vi "Sequence.AddVariables.vi"(8 "error in (no error)":errorcluster, 10 "Channels":T1[](array[typedef]), 11 "Sequence":refnum<k24>) -> (0 "error out":errorcluster, 3 "Sequence out":refnum<k24>)   [LabVIEW 2013, in "Simple Sequence Editor.lvlib"]
uses:
  Simple Sequence Editor.lvlib
  NationalInstruments.VeriStand.RealTimeSequenceDefinitionApi
  Types/ChannelProperties.ctl
  Constants.vi
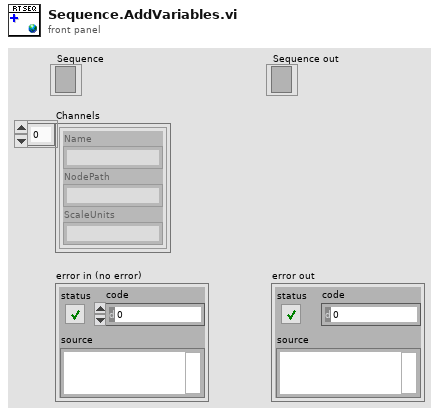
[diagram p1: front panel]
types:
  T1 = typedef "Simple Sequence Editor.lvlib/ChannelProperties.ctl" = cluster{"Name":string, "NodePath":string, "ScaleUnits":string}
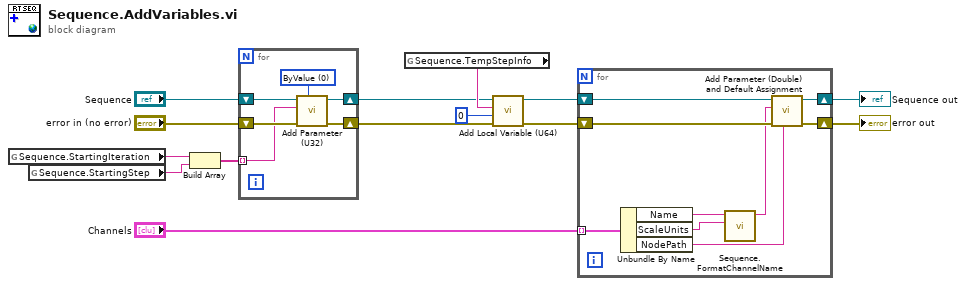
[diagram p0: block diagram]
diagram:
  n1 = global read "Constants.vi" "Sequence.StartingIteration"() -> (w11:string)
  n2 = global read "Constants.vi" "Sequence.StartingStep"() -> (w12:string)
  n3 = Build Array(w11, w12) -> (w13:string[])
  n4 = for {
    shift-right: [w20] -> w6
    shift-left: "error in (no error)" -> [w17]
    shift-right: [w19] -> w8
    shift-left: "Sequence" -> [w18]
    tunnel: w13 -> [w15] mode=indexing
    w16 = 0 items=["ByValue", "ByReference"] ("Evaluation Method (ByReference)")
    n5 = call "Add Parameter (U32).vi"("Evaluation Method (ByReference)"=w16, "error in (no error)"=w17, "Identifier"=w15, "Sequence Ref in"=w18) -> ("error out"=w20:errorcluster, "Sequence Ref out"=w19:refnum<k24>)  [unwired: 6 in]
  }
  n6 = global read "Constants.vi" "Sequence.TempStepInfo"() -> (w14:string)
  n7 = call "Add Local Variable (U64).vi"("error in (no error)"=w6, "Value"=u64 0, "Identifier"=w14, "Sequence Ref in"=w8) -> ("error out"=w7:errorcluster, "Sequence Ref out"=w9:refnum<k24>)  [unwired: 6 in]
  n8 = for {
    tunnel: "Channels" -> [w29] mode=indexing
    shift-right: [w22] -> w2
    shift-left: w7 -> [w25]
    shift-right: [w21] -> w3
    shift-left: w9 -> [w26]
    n9 = Unbundle By Name(w29) -> ("Name"=w28:string, "ScaleUnits"=w27:string, "NodePath"=w23:string)
    n10 = call "Sequence.FormatChannelName.vi"("ScaleUnits"=w27, "Name"=w28) -> ("String"=w24:string)  [unwired: 9 in]
    n11 = call "Add Parameter (Double) and Default Assignment.vi"("Default Assignment"=w23, "error in (no error)"=w25, "Identifier"=w24, "Sequence Ref in"=w26) -> ("error out"=w22:errorcluster, "Sequence Ref out"=w21:refnum<k24>)  [unwired: 6 in]
  }
  "Sequence out" <- w3
  "error out" <- w2
